vi "ukol3.vi"() -> ()   [LabVIEW 2022 SP3]
panel:
  out "appended array":string[][](array[string])
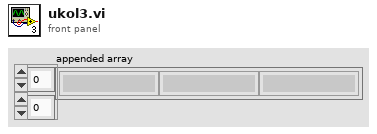
[diagram p1: front panel]
types:
  T1 = enum16{"open", "replace", "create", "open or create", "replace or create", "replace or create with confirmation"}
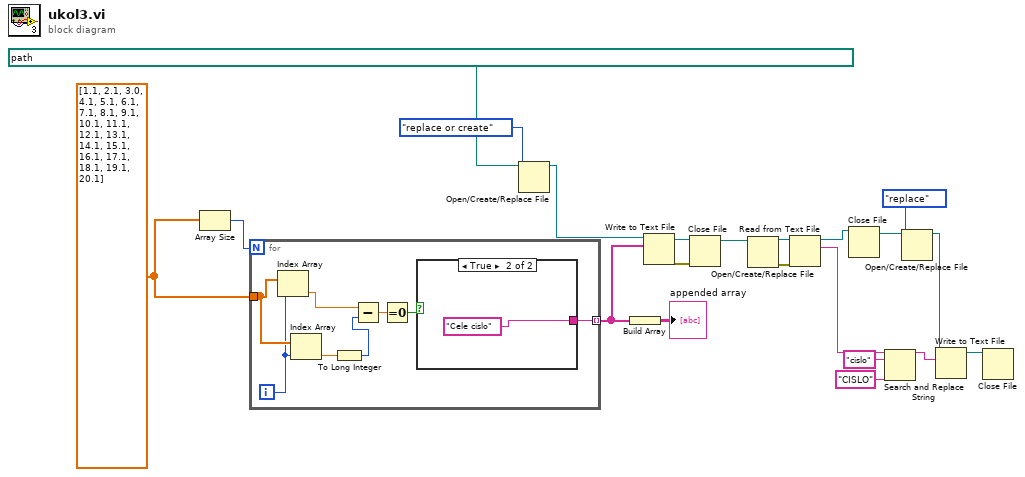
[diagram p0: block diagram]
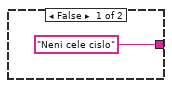
[diagram p2: hidden frame]
diagram:
  w3 = dbl[] [1.1, 2.1, 3.0, 4.1, 5.1, 6.1, 7.1, 8.1, 9.1, 10.1, 11.1, 12.1, 13.1, 14.1, 15.1, 16.1, 17.1, 18.1, 19.1, 20.1]
  n1 = Array Size(array=w3) -> (size(s)=w4:i32)
  n2 = for {
    N: w4 -> [_]
    tunnel: [w29] -> w2 mode=indexing
    tunnel: w3 -> [w28]
    i -> [w27]
    n3 = Index Array(array=w28, index=w27) -> (element=w24:dbl)
    n4 = Index Array(array=w28, index=w27) -> (element=w26:dbl)
    n5 = To Long Integer(number=w26) -> (32bit integer=w25:i32)
    n6 = Subtract(x=w24, y=w25) -> (x-y=w23:dbl)
    n7 = Equal To 0?(x=w23) -> (x = 0?=w22:bool)
    n8 = case shown="True" w22 {
      tunnel: ["Neni cele cislo" "Cele cislo"] -> w29
      frame False {
      }
      frame True {
      }
    }
  }
  n9 = Open/Create/Replace File(file path (use dialog)=path "C:/Users/mmara/OneDrive/Dokumenty/Magisterské studium/Letní semestr/Elektronické měřící systémy/Projekt/EMS_projekt/State machine/emscv7/data.txt", operation (0:open)=T1."replace or create") -> (refnum out=w21:refnum<file>)  [unwired: 4 in, 2 out]
  n10 = Build Array(w2) -> (→"appended array":string[][])
  n11 = Write to Text File(file (use dialog)=w21, text=w2) -> (refnum out=w19:refnum<file>, error out=w18:errorcluster)  [unwired: 2 in, 1 out]
  n12 = Close File(refnum=w19, error in=w18) -> (path=w17:path)  [unwired: 1 out]
  n13 = Open/Create/Replace File(file path (use dialog)=w17) -> (refnum out=w15:refnum<file>, error out=w16:errorcluster)  [unwired: 5 in, 1 out]
  n14 = Read from Text File(file (use dialog)=w15, error in=w16) -> (refnum out=w10:refnum<file>, text=w14:string)  [unwired: 2 in, 2 out]
  n15 = Close File(refnum=w10) -> (path=w9:path)  [unwired: 1 in, 1 out]
  n16 = Search and Replace String(input string=w14, search string="cislo", replace string="CISLO" ("replace string (\"\")")) -> (result string=w11:string)  [unwired: 5 in, 3 out]
  n17 = Open/Create/Replace File(file path (use dialog)=w9, operation (0:open)=T1."replace") -> (refnum out=w7:refnum<file>)  [unwired: 4 in, 2 out]
  n18 = Write to Text File(file (use dialog)=w7, text=w11) -> (refnum out=w6:refnum<file>)  [unwired: 2 in, 2 out]
  n19 = Close File(refnum=w6) -> ()  [unwired: 1 in, 2 out]
